vi "pannel-to-str.vi"(11 "pannel":T1(array[cluster]) {"ID" format="%02x"}) -> (3 "字符串":string)   [LabVIEW 2019]
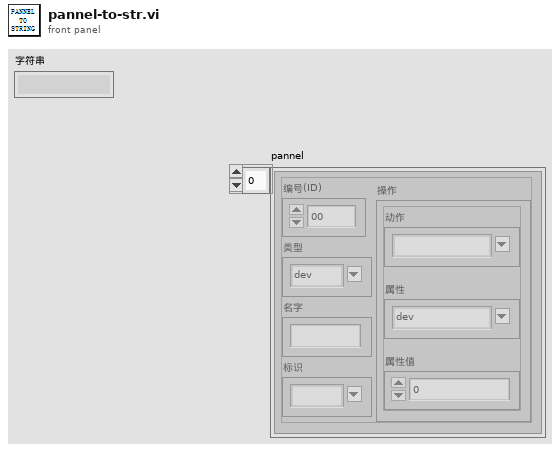
[diagram p1: front panel]
types:
  T1 = cluster{"ID":u8, "type":string, "flag":string, "name":string, "Act":cluster{"Attribute":string, "Action":string, "Value":dbl}}[]
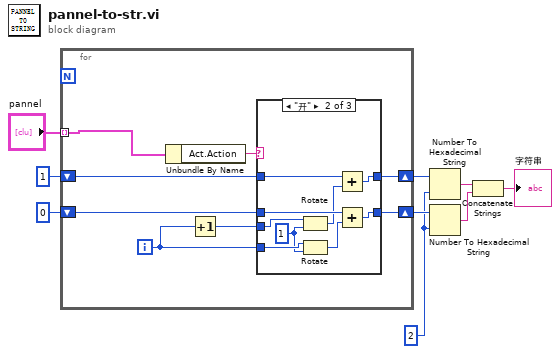
[diagram p0: block diagram]
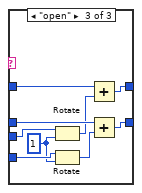
[diagram p3: hidden frame]
diagram:
  w4 = i16 2 ("宽度(-)")
  n1 = for {
    tunnel: "pannel" -> [w10] mode=indexing
    shift-right: [w16] -> w6
    shift-left: i16 0 -> [w15]
    shift-right: [w12] -> w5
    shift-left: i16 1 -> [w11]
    i -> [w14]
    n2 = Unbundle By Name(w10) -> ("Act.Action"=w17:string)
    n3 = Increment(x=w14) -> (x+1=w13:i32)
    n4 = case shown="\"开\"" w17 {
      tunnel: w14 -> [_ w27 w36]
      tunnel: [w19 w26 w35] -> w16
      tunnel: w15 -> [w19 w25 w34]
      tunnel: w13 -> [_ w23 w32]
      tunnel: [w18 w21 w30] -> w12
      tunnel: w11 -> [w18 w20 w29]
      frame "关", Default {
      }
      frame "开" {
        w24 = i16 1 ("y")
        n5 = Rotate(1:w24, 2:w23) -> (0:w22:i16)
        n6 = Rotate(1:w24, 2:w27) -> (0:w28:i16)
        n7 = Add(x=w20, y=w22) -> (x+y=w21:i16)
        n8 = Add(x=w25, y=w28) -> (x+y=w26:i16)
      }
      frame "open" {
        w33 = i16 1 ("y")
        n9 = Rotate(1:w33, 2:w32) -> (0:w31:i16)
        n10 = Rotate(1:w33, 2:w36) -> (0:w37:i16)
        n11 = Add(x=w29, y=w31) -> (x+y=w30:i16)
        n12 = Add(x=w34, y=w37) -> (x+y=w35:i16)
      }
    }
  }
  n13 = Number To Hexadecimal String(1:w4, 2:w5) -> (0:w3:string)
  n14 = Number To Hexadecimal String(1:w4, 2:w6) -> (0:w2:string)
  n15 = Concatenate Strings(w3, w2) -> (→"字符串":string)
